vi "GPIB Device.vi"(0 "Point #":i32) -> (1 "GPIB Data Out":dbl[](array[numeric]) format="%.2e", 2 "Stop Out":bool)   [LabVIEW 2025]
doc: "VI which calls the appropriate GPIB routines for a variety of instruments.\nScott Hannahs, NHMFL-FSU, Nov. 1993\nAuthor: Scott Hannahs <sth@magnet.fsu.edu>\n\nThis software is licensed for use under the “MIT License\"\nCopyright (c) 2025 Scott Hannahs, sth@sth@magnet.sthnet.net\n\nPermission is hereby granted, free of charge, to any person obtaining a copy of this software and associated documentation files (the \"Software\"), to deal in the Software without restriction, including without limitation the rights to use, copy, modify, merge, publish, distribute, sublicense, and/or sell copies of the Software, and to permit persons to whom the Software is furnished to do so, subject to the following conditions: The above copyright notice and this permission notice shall be included in all copies or substantial portions of the Software.\n\nTHE SOFTWARE IS PROVIDED \"AS IS\", WITHOUT WARRANTY OF ANY KIND, EXPRESS OR IMPLIED, INCLUDING BUT NOT LIMITED TO THE WARRANTIES OF MERCHANTABILITY, FITNESS FOR A PARTICULAR PURPOSE AND NONINFRINGEMENT. IN NO EVENT SHALL THE AUTHORS OR COPYRIGHT HOLDERS BE LIABLE FOR ANY CLAIM, DAMAGES OR OTHER LIABILITY, WHETHER IN AN ACTION OF CONTRACT, TORT OR OTHERWISE, ARISING FROM, OUT OF OR IN CONNECTION WITH THE SOFTWARE OR THE USE OR OTHER DEALINGS IN THE SOFTWARE."
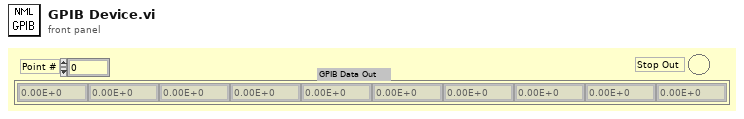
[diagram p1: front panel]
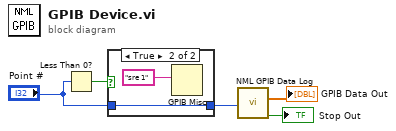
[diagram p0: block diagram]
diagram:
  n1 = Less Than 0?(x="Point #") -> (x < 0?=w3:bool)
  n2 = case shown="True" w3 {
    tunnel: [w6 w7] -> w1
    tunnel: "Point #" -> [w6 w7]
    frame False {
    }
    frame True {
      n3 = GPIB Misc(0:"sre 1") -> ()  [unwired: 1 in, 3 out]
    }
  }
  n4 = call "NML GPIB Data Log.vi"("Point #"=w1) -> ("GPIB Data"=→"GPIB Data Out":dbl[], "Stop"=→"Stop Out":bool)
